vi "Build Type Specialization Value.vi"(11 "error in (no error)":errorcluster) -> (4 "Type Specialization":T1(array[cluster]), 15 "error out":errorcluster)   [LabVIEW 2021, in "Migrator.lvlib"]
uses:
  Migrator.lvlib
  Migrator Reusables/Migrator Reusables.lvlib
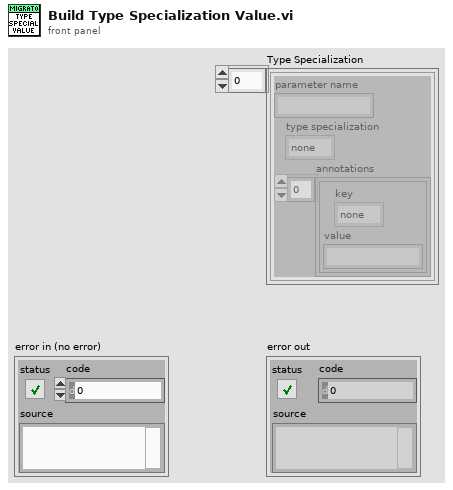
[diagram p1: front panel]
types:
  T1 = cluster{"parameter name":string, "type specialization":enum16{"none", "pin", "path", "enum"}, "annotations":cluster{"key":enum16{"none", "pin.instrument_type", "enum.values"}, "value":string}[]}[]
  T2 = cluster{"parameter name":string, "type specialization":enum16{"none", "pin", "path", "enum", "ioresource"}, "annotations":cluster{"key":enum16{"none", "pin.instrument_type", "enum.values", "ioresource.instrument_type"}, "value":string}[]}
  T3 = cluster{"parameter name":string, "type specialization":enum16{"none", "pin", "path", "enum"}, "annotations":cluster{"key":enum16{"none", "pin.instrument_type", "enum.values"}, "value":string}[]}
  T4 = cluster{"key":enum16{"none", "pin.instrument_type", "enum.values"}, "value":string}[]
  T5 = enum16{"none", "pin.instrument_type", "enum.values"}
  T6 = cluster{"key":enum16{"none", "pin.instrument_type", "enum.values"}, "value":string}
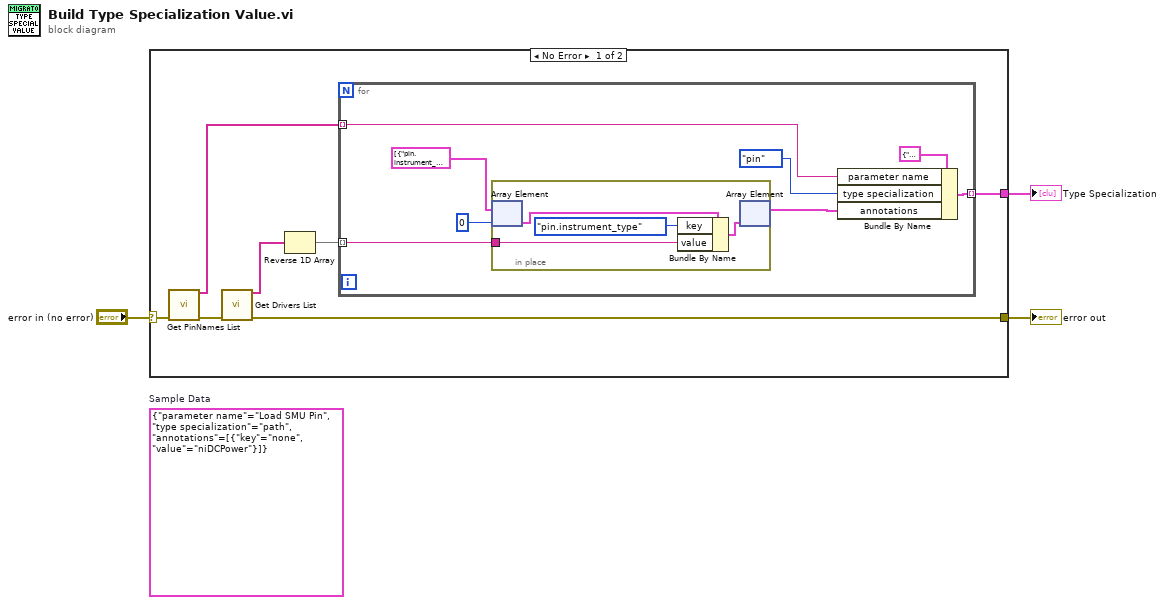
[diagram p0: block diagram]
diagram:
  (unwired) T2 {"parameter name"="Load SMU Pin", "type specialization"=enum."path", "annotations"=[{"key"=enum."none", "value"="niDCPower"}]}  # Sample Data
  n1 = case shown="No Error" "error in (no error)" {
    selector: "error in (no error)" -> [w8 w23]
    tunnel: [w10 w23] -> w3
    tunnel: [w5 _] -> w1
    frame No Error {
      n2 = call "Get PinNames List.vi"("error in (no error)"=w8) -> ("PinNames Label"=w6:string[], "error out"=w7:errorcluster)  [unwired: 13 in]
      n3 = call "Get Drivers List.vi"("error in (no error)"=w7) -> ("Drivers List Out"=w9:string[], "error out"=w10:errorcluster)  [unwired: 9 in, 4 out]
      n4 = Reverse 1D Array(array=w9) -> (reversed array=w4:string[])
      n5 = for {
        tunnel: [w18] -> w5 mode=indexing
        tunnel: w4 -> [w14] mode=indexing
        tunnel: w6 -> [w11] mode=indexing
        n6 = in-place {
          in-place-border: w14 -> [w19]
          n7 = in-place-array #1(T4 [{"key"=enum."pin.instrument_type", "value"=""}] ("annotations"), 0) -> (w22:T6)
          n8 = Bundle By Name(cluster=w22, "key"=T5."pin.instrument_type", "value"=w19) -> (w20:T6)
          n9 = in-place-array #1(w20) -> (w12:T4)  [unwired: 1 out]
        }
        n10 = Bundle By Name(cluster=T3 {"parameter name"="", "type specialization"=enum."none", "annotations"=[]} ("Type Specializations"), "parameter name"=w11, "type specialization"=enum16{"none", "pin", "path", "enum"}."pin", "annotations"=w12) -> (w18:T3)
      }
    }
    frame Error {
    }
  }
  "error out" <- w3
  "Type Specialization" <- w1
